vi "read tdms.vi"() -> ()   [LabVIEW 2011]
panel:
  in  "stop":bool
  out "error out":errorcluster
  in  "CCDs":string[](array[string])=["L4_TREXpass1", "L5_TREXPass2", "L6_TREXpass3", "L7_TREXPass4", "L8_M10Leak", "B1_TelInput", "B2_TelLens1", "B5_CompressorOut", "", "", "", ""]
  in  "file path":path
  out "CCD 1":cluster{timestamp[], dbl[]}[](graph)
  out "CCD 2":cluster{timestamp[], dbl[]}[](graph)
  out "CCD 3":cluster{timestamp[], dbl[]}[](graph)
  out "CCD 4":cluster{timestamp[], dbl[]}[](graph)
  out "CCD 5":cluster{timestamp[], dbl[]}[](graph)
  out "CCD 6":cluster{timestamp[], dbl[]}[](graph)
  out "CCD 7":cluster{timestamp[], dbl[]}[](graph)
  out "CCD 8":cluster{timestamp[], dbl[]}[](graph)
  out "CCD 11":cluster{timestamp[], dbl[]}[](graph)
  out "CCD 9":cluster{timestamp[], dbl[]}[](graph)
  out "CCD 12":cluster{timestamp[], dbl[]}[](graph)
  out "CCD 10":cluster{timestamp[], dbl[]}[](graph)
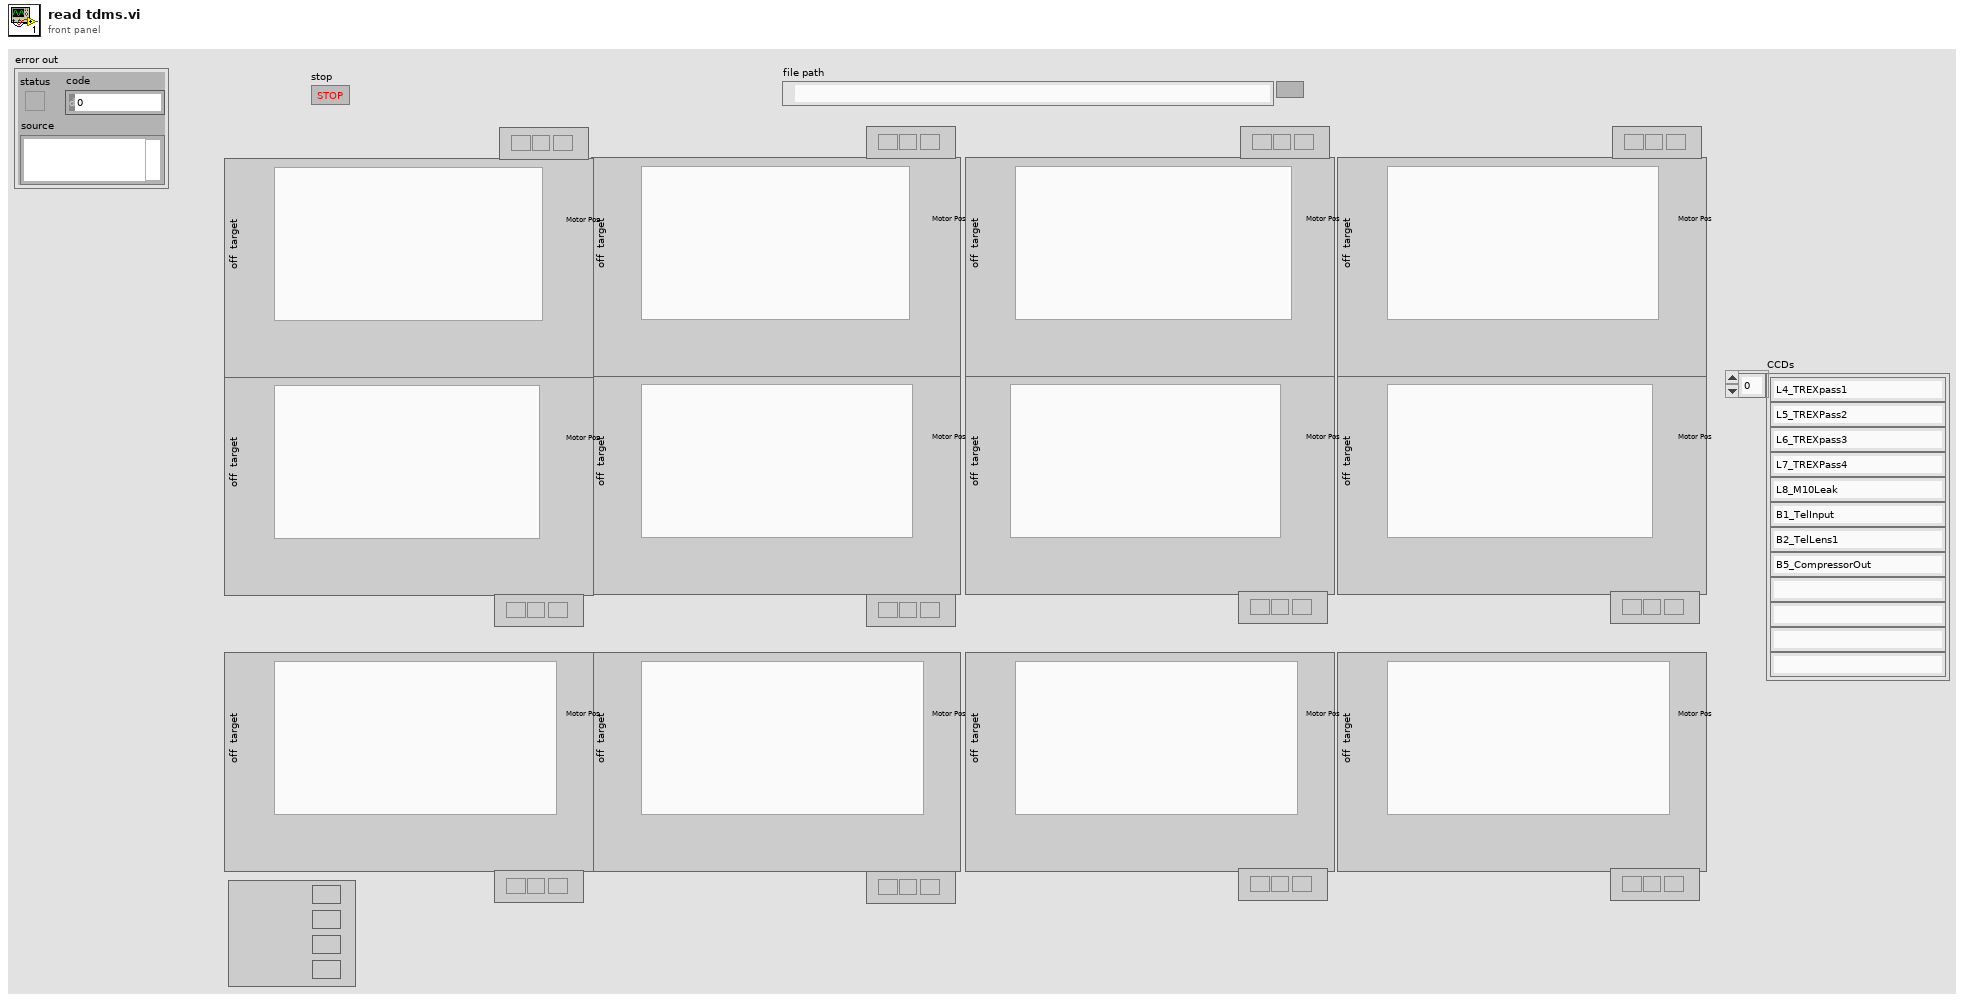
[diagram p1: front panel]
types:
  T1 = cluster{"appended array":timestamp[], "appended array":dbl[]}
  T2 = cluster{"appended array":timestamp[], "appended array":dbl[]}[]
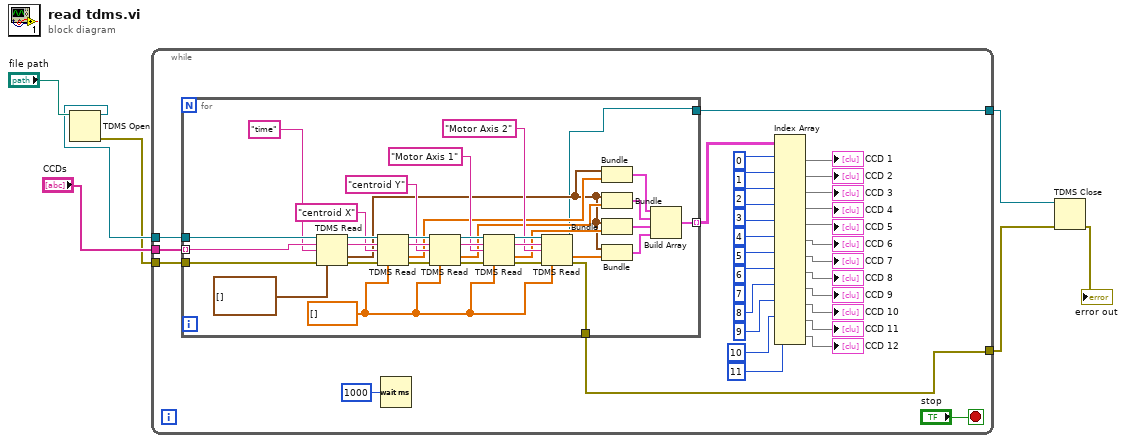
[diagram p0: block diagram]
diagram:
  n1 = TDMS Open(11:"file path") -> (0:w4:errorcluster, 3:w6:refnum<k34>)  [unwired: 5 in]
  n2 = while {
    tunnel: w6 -> [w27]
    tunnel: "CCDs" -> [w26]
    tunnel: w4 -> [w25]
    tunnel: [w11] -> w3
    tunnel: [w10] -> w2
    stop <- "stop" stop-if-true
    n3 = for {
      tunnel: w27 -> [w73]
      tunnel: w26 -> [w72] mode=indexing
      tunnel: w25 -> [w56]
      tunnel: [w42] -> w24 mode=indexing
      tunnel: [w41] -> w10
      tunnel: [w40] -> w11
      w57 = dbl[] [] ("appended array")
      n4 = TDMS Read(0:w73, 5:w72, 7:"time", 11:w56, 12:timestamp[] [] ("appended array")) -> (4:w71:refnum<k34>, 6:w67:string, 10:w48:timestamp[], 15:w55:errorcluster)  [unwired: 3 in, 2 out]
      n5 = TDMS Read(0:w71, 5:w67, 7:"centroid X", 11:w55, 12:w57) -> (4:w70:refnum<k34>, 6:w66:string, 10:w51:dbl[], 15:w54:errorcluster)  [unwired: 3 in, 2 out]
      n6 = TDMS Read(0:w70, 5:w66, 7:"centroid Y", 11:w54, 12:w57) -> (4:w69:refnum<k34>, 6:w65:string, 10:w50:dbl[], 15:w53:errorcluster)  [unwired: 3 in, 2 out]
      n7 = TDMS Read(0:w69, 5:w65, 7:"Motor Axis 1", 11:w53, 12:w57) -> (4:w68:refnum<k34>, 6:w64:string, 10:w49:dbl[], 15:w52:errorcluster)  [unwired: 3 in, 2 out]
      n8 = TDMS Read(0:w68, 5:w64, 7:"Motor Axis 2", 11:w52, 12:w57) -> (4:w40:refnum<k34>, 10:w47:dbl[], 15:w41:errorcluster)  [unwired: 3 in, 3 out]
      n9 = Bundle("appended array"=w48, "appended array"=w51) -> (w46:T1)  [unwired: 1 in]
      n10 = Bundle("appended array"=w48, "appended array"=w50) -> (w45:T1)  [unwired: 1 in]
      n11 = Bundle("appended array"=w48, "appended array"=w49) -> (w44:T1)  [unwired: 1 in]
      n12 = Bundle("appended array"=w48, "appended array"=w47) -> (w43:T1)  [unwired: 1 in]
      n13 = Build Array(w46, w45, w44, w43) -> (w42:T2)
    }
    n14 = Wait (ms)(milliseconds to wait=u32 1000) -> ()  [unwired: 1 out]
    n15 = Index Array(array=w24, index (row) #1=0 ("index (row)"), index (row) #2=1 ("index (row)"), index (row) #3=2 ("index (row)"), index (row) #4=3 ("index (row)"), index (row) #5=4 ("index (row)"), index (row) #6=5 ("index (row)"), index (row) #7=6 ("index (row)"), index (row) #8=7 ("index (row)"), index (row) #9=8 ("index (row)"), index (row) #10=9 ("index (row)"), index (row) #11=10 ("index (row)"), index (row) #12=11 ("index (row)")) -> (element #1=→"CCD 1":T2, element #2=→"CCD 2":T2, element #3=→"CCD 3":T2, element #4=→"CCD 4":T2, element #5=→"CCD 5":T2, element #6=→"CCD 6":T2, element #7=→"CCD 7":T2, element #8=→"CCD 8":T2, element #9=→"CCD 9":T2, element #10=→"CCD 10":T2, element #11=→"CCD 11":T2, element #12=→"CCD 12":T2)  [unwired: 12 in]
  }
  n16 = TDMS Close(8:w2, 11:w3) -> (0:→"error out":errorcluster)  [unwired: 1 out]
